vi "Connect Cells.vi"(9 "To":T1, 10 "From":T1, 11 "Adjacency In":T2[][](array[typedef])) -> (3 "Adjacency":T2[][](array[typedef]))   [LabVIEW 2020, in "Maze.lvlib" / "MazeGen.lvclass"]
uses:
  MazeGen.lvclass
  Adjacency.ctl
  Position.ctl
  Maze.lvlib
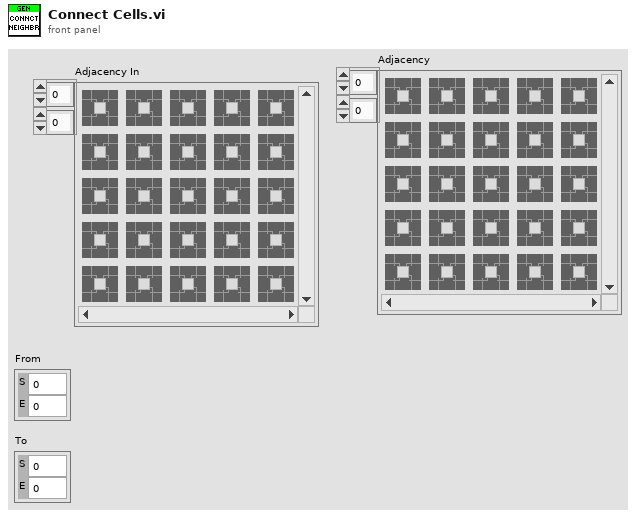
[diagram p1: front panel]
types:
  T1 = typedef "Maze.lvlib/Position.ctl" = cluster{"S":i32, "E":i32}
  T2 = typedef "Maze.lvlib/Adjacency.ctl" = cluster{"E":bool, "N":bool, "W":bool, "S":bool, "Goal":bool, "Start":bool}
  T3 = typedef "Maze.lvlib/Direction.ctl" = enum8{"East", "North", "West", "South"}
  T4 = cluster{"Adjacency[0]":bool, "Adjacency[1]":bool, "Adjacency[2]":bool, "Adjacency[3]":bool, "Adjacency[4]":bool, "Adjacency[5]":bool}
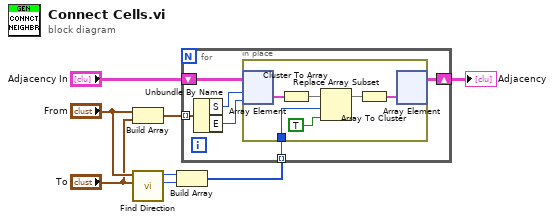
[diagram p0: block diagram]
diagram:
  n1 = Build Array("From", "To") -> (w1:T1[])
  n2 = call "Find Direction.vi"("To"="To", "From"="From") -> ("Opposite"=w3:T3, "Direction"=w4:T3)  [unwired: 7 in, 1 out]
  n3 = Build Array(w4, w3) -> (w2:T3[])
  n4 = for {
    shift-right: [w11] -> w7
    shift-left: "Adjacency In" -> [w14]
    tunnel: w2 -> [w10] mode=indexing
    tunnel: w1 -> [w9] mode=indexing
    n5 = Unbundle By Name(w9) -> ("S"=w13:i32, "E"=w12:i32)
    n6 = in-place {
      in-place-border: w10 -> [w18]
      n7 = in-place-array #1(w14, w13, w12) -> (w20:T2)
      n8 = Cluster To Array(cluster=w20) -> (array=w19:bool[])
      n9 = Replace Array Subset(array=w19, new element=TRUE ("new element/subarray"), index=w18) -> (w16:bool[])
      n10 = Array To Cluster(array=w16) -> (cluster=w15:T4)
      n11 = in-place-array #1(w15) -> (w11:T2[][])  [unwired: 2 out]
    }
  }
  "Adjacency" <- w7
